vi "Get MathFunction Name.vi"(8 "error in (no error)":errorcluster, 11 "Calculator in":refnum<class "MathFunction.lvclass">) -> (0 "error out":errorcluster, 2 "MathFunction Name":string, 3 "Calculator out":refnum<class "MathFunction.lvclass">)   [LabVIEW 2019, in "lv-classprovidershell-example.lvlib" / "MathFunction.lvclass"]
uses:
  MathFunction.lvclass
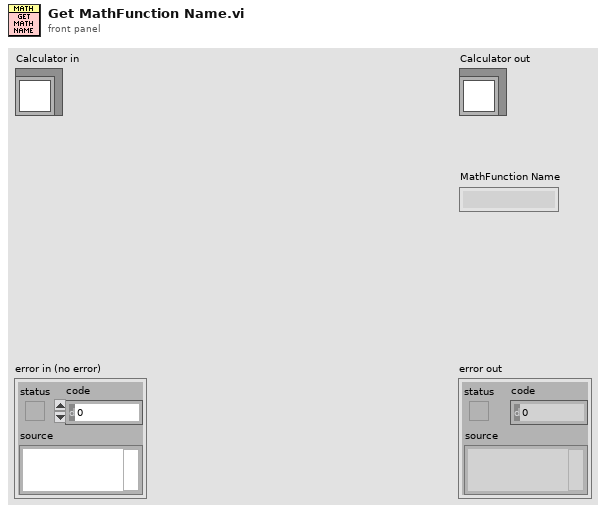
[diagram p1: front panel]
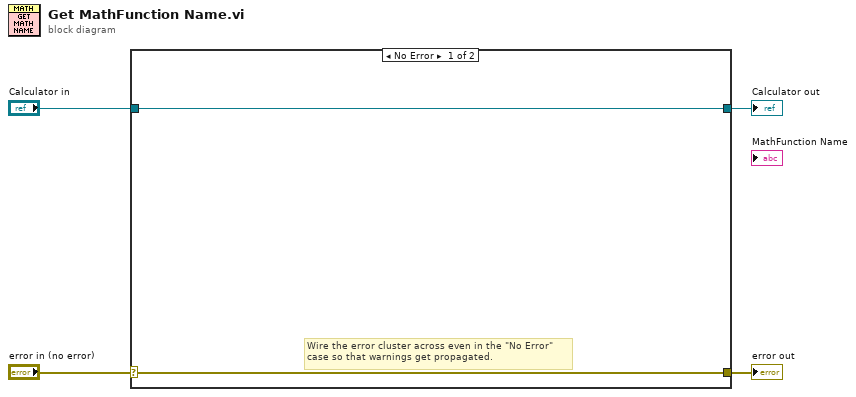
[diagram p0: block diagram]
diagram:
  n1 = case shown="No Error" "error in (no error)" {
    selector: "error in (no error)" -> [w5 w8]
    tunnel: [w5 w8] -> w3
    tunnel: [w6 w7] -> w1
    tunnel: "Calculator in" -> [w6 w7]
    frame No Error {
      # "Wire the error cluster across even in the \"No Error\"\ncase so that warnings get propagated."
    }
    frame Error {
    }
  }
  "error out" <- w3
  "Calculator out" <- w1
